vi "SysIdRoutine_Quasistatic.vi"(6 "reset?":bool, 10 "direction":enum16{"kForward", "kReverse"}(ring), 11 "in SysIdRoutine":T3={"m_config"={"m_timeout_Sec"=10.0, "m_stepVoltage_Volt"=7.0, "m_rampRate_V/S"=1.0}, "m_mechanism"={"m_drive_volts"=0.0, "m_log"=[], "m_name"=""}, "m_outputVolts"=0.0, "m_recordState"=enum."kNone", "timer"={"StartTime"=0.0, "Accumulated TIme"=0.0, "Running"=FALSE, "semaphore"=refnum}} {"timer"."Accumulated TIme" format="%13.5p"; "timer"."StartTime" format="%13.5p"}) -> (0 "Expired":bool, 1 "CurrentTimer":dbl, 2 "outputVolts":dbl, 3 "out SysIdRoutine":T3={"m_config"={"m_timeout_Sec"=10.0, "m_stepVoltage_Volt"=7.0, "m_rampRate_V/S"=1.0}, "m_mechanism"={"m_drive_volts"=0.0, "m_log"=[], "m_name"=""}, "m_outputVolts"=0.0, "m_recordState"=enum."kNone", "timer"={"StartTime"=0.0, "Accumulated TIme"=0.0, "Running"=FALSE, "semaphore"=refnum}} {"timer"."Accumulated TIme" format="%13.5p"; "timer"."StartTime" format="%13.5p"})   [LabVIEW 2023]
uses:
  <vilib>/Rock Robotics/WPI/ThirdParty/JAS_Junk/TrajLib/TypeDef/TIMER.ctl
  <vilib>/Utility/semaphor.llb/Obtain Semaphore Reference.vi
  <vilib>/Rock Robotics/WPI/ThirdParty/JAS_Junk/TrajLib/Timer_Reset.vi
  <vilib>/Rock Robotics/WPI/ThirdParty/JAS_Junk/TrajLib/Trajectory_Library.lvlib
panel:
  out "outputSign":dbl
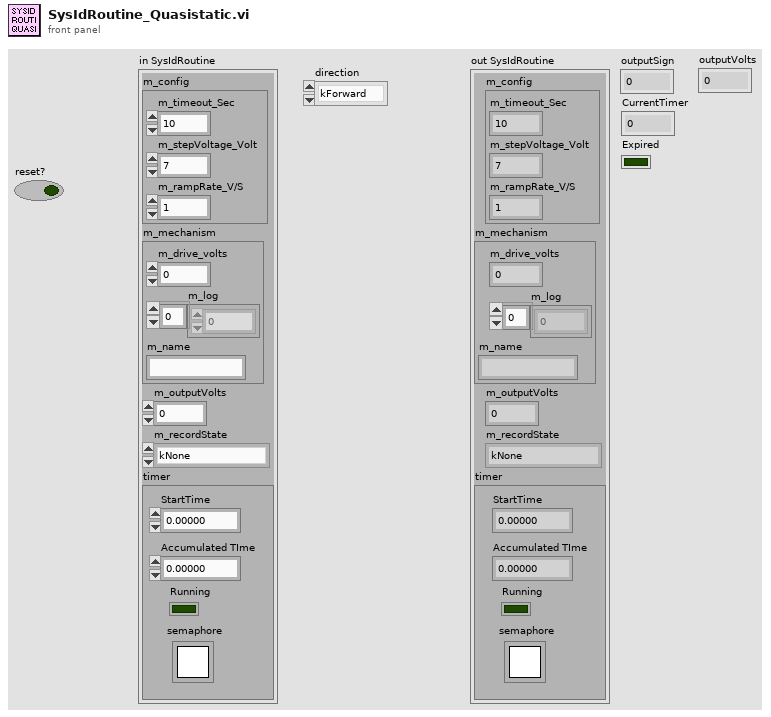
[diagram p1: front panel]
types:
  T1 = typedef "Trajectory_Library.lvlib/TIMER.ctl" = cluster{"StartTime":dbl, "Accumulated TIme":dbl, "Running":bool, "semaphore":T2}
  T2 = typedef "Semaphore RefNum" = refnum<k1>
  T3 = cluster{"m_config":cluster{"m_timeout_Sec":dbl, "m_stepVoltage_Volt":dbl, "m_rampRate_V/S":dbl}, "m_mechanism":cluster{"m_drive_volts":dbl, "m_log":u8[], "m_name":string}, "m_outputVolts":dbl, "m_recordState":enum16{"kQuasistaticForward", "kQuasistaticReverse", "kDynamicForward", "kDynamicReverse", "kNone"}, "timer":T1}
  T4 = enum16{"big-endian, network order", "native, host order", "little-endian"}
  T5 = enum16{"kQuasistaticForward", "kQuasistaticReverse", "kDynamicForward", "kDynamicReverse", "kNone"}
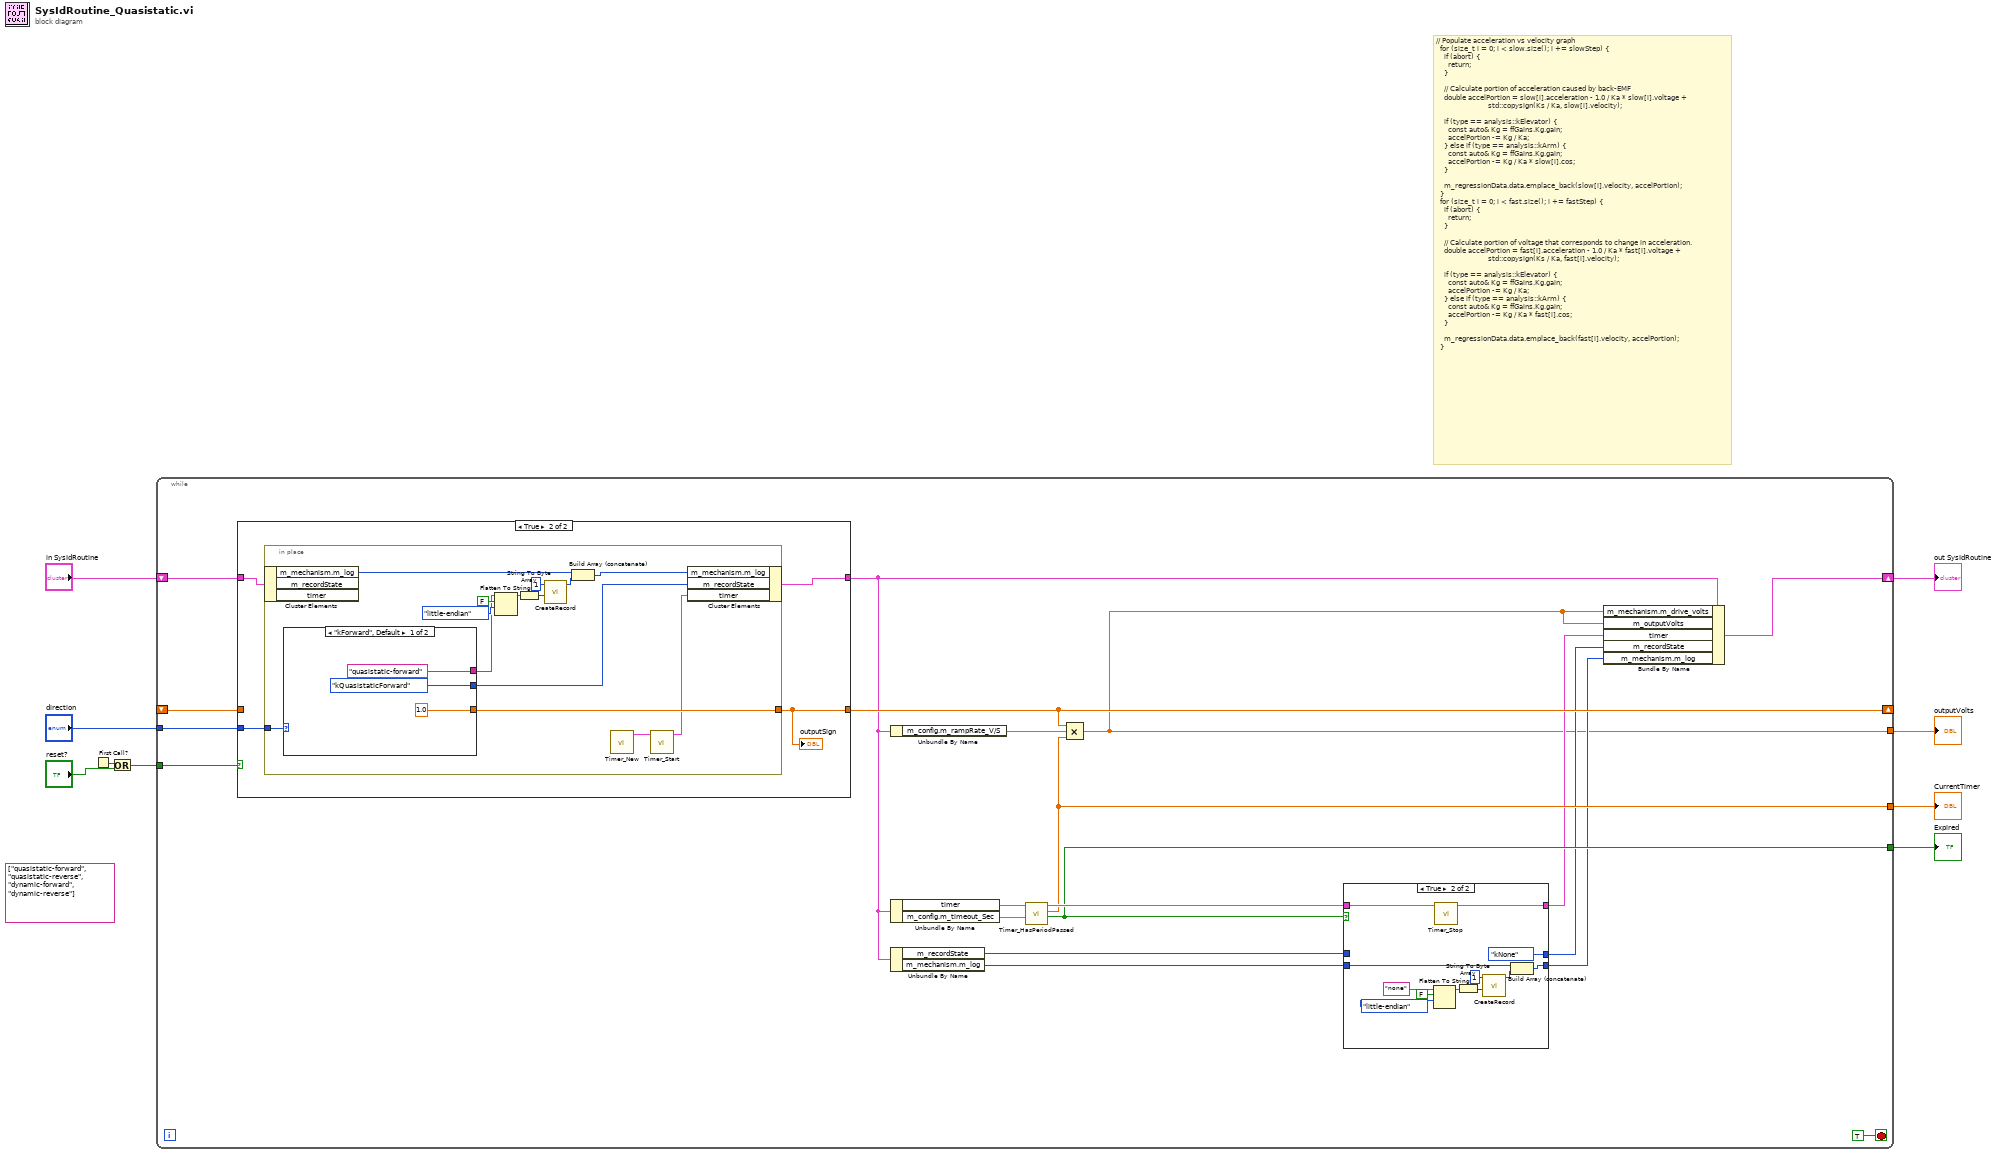
[diagram p0: block diagram]
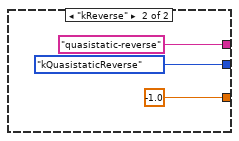
[diagram p3: hidden frame]
diagram:
  (unwired) string[] ["quasistatic-forward", "quasistatic-reverse", "dynamic-forward", "dynamic-reverse"]
  # "// Populate acceleration vs velocity graph\n  for (size_t i = 0; i < slow.size(); i += slowStep) {\n    if (abort) {\n      return;\n    }\n\n    // Calculate portion of acceleration caused by back-EMF\n    double accelPortion = slow[i].acceleration - 1.0 / Ka * slow[i].voltage +\n                          std::copysign(Ks / Ka, slow[i].velocity);\n\n    if (type == analysis::kElevator) {\n      const auto& Kg = ffGains.Kg.gain;\n      accelPortion -= Kg / Ka;\n    } else if (type == analysis::kArm) {\n      const auto& Kg = ffGains.Kg.gain;\n      accelPortion -= Kg / Ka * slow[i].cos;\n    }\n\n    m_regressionData.data.emplace_back(slow[i].velocity, accelPortion);\n  }\n  for (size_t i = 0; i < fast.size(); i += fastStep) {\n    if (abort) {\n      return;\n    }\n\n    // Calculate portion of voltage that corresponds to change in acceleration.\n    double accelPortion = fast[i].acceleration - 1.0 / Ka * fast[i].voltage +\n                          std::copysign(Ks / Ka, fast[i].velocity);\n\n    if (type == analysis::kElevator) {\n      const auto& Kg = ffGains.Kg.gain;\n      accelPortion -= Kg / Ka;\n    } else if (type == analysis::kArm) {\n      const auto& Kg = ffGains.Kg.gain;\n      accelPortion -= Kg / Ka * fast[i].cos;\n    }\n\n    m_regressionData.data.emplace_back(fast[i].velocity, accelPortion);\n  }"
  n1 = First Call?() -> (First Call?: T/F=w4:bool)
  n2 = Or(x=w4, y="reset?") -> (x .or. y?=w2:bool)
  n3 = while {
    tunnel: "direction" -> [w29]
    shift-right: [w23] -> w7
    shift-left: "in SysIdRoutine" -> [w28]
    tunnel: [w21] -> w6
    tunnel: [w20] -> w5
    shift-right: [w19] -> _
    shift-left: _ -> [w18]
    tunnel: w2 -> [w12]
    tunnel: [w11] -> w1
    stop <- TRUE stop-if-true
    n4 = case shown="True" w12 {
      tunnel: w29 -> [_ w35]
      tunnel: w28 -> [w31 w34]
      tunnel: [w30 w33] -> w19
      tunnel: [w31 w32] -> w17
      tunnel: w18 -> [w30 _]
      frame False {
      }
      frame True {
        n5 = in-place {
          in-place-border: w35 -> [w49]
          in-place-border: [w47] -> w33
          n6 = in-place-cluster #1(w34) -> ("m_mechanism.m_log"=w40:u8[])  [unwired: 2 out]
          n7 = case shown="\"kForward\", Default" w49 {
            tunnel: [T5."kQuasistaticForward" ("m_recordState") T5."kQuasistaticReverse" ("m_recordState")] -> w48
            tunnel: [1.0 -1.0] -> w47
            tunnel: ["quasistatic-forward" ("String") "quasistatic-reverse" ("String")] -> w38
            frame "kForward", Default {
            }
            frame "kReverse" {
            }
          }
          n8 = Flatten To String(anything=w38, prepend array or string size? (T)=FALSE, byte order (0:big-endian, network order)=T4."little-endian") -> (data string=w44:string)  [unwired: 1 in, 2 out]
          n9 = String To Byte Array(string=w44) -> (unsigned byte array=w45:u8[])
          n10 = call "CreateRecord.vi"("payload data (little endian)"=w45, "entry ID"=1) -> ("record"=w46:u8[])  [unwired: 9 in]
          n11 = Build Array (concatenate)(w40, w46) -> (w39:u8[])
          n12 = call <vilib>:"Timer_New.vi"() -> ("TIMER"=w37:T1)  [unwired: 11 in]
          n13 = call <vilib>:"Timer_Start.vi"("in Timer"=w37) -> ("out Timer"=w36:T1)  [unwired: 10 in]
          n14 = in-place-cluster #1("m_mechanism.m_log"=w39, "m_recordState"=w48, "timer"=w36) -> (w32:T3)
        }
        "outputSign" <- w33
      }
    }
    n15 = Unbundle By Name(w17) -> ("m_config.m_rampRate_V/S"=w24:dbl)
    n16 = Unbundle By Name(w17) -> ("timer"=w26:T1, "m_config.m_timeout_Sec"=w25:dbl)
    n17 = Unbundle By Name(w17) -> ("m_recordState"=w15:T5, "m_mechanism.m_log"=w10:u8[])
    n18 = call <vilib>:"Timer_HasPeriodPassed.vi"("Period"=w25, "in Timer"=w26) -> ("Expired"=w20:bool, "CurrentTImer"=w21:dbl, "out Timer"=w27:T1)  [unwired: 7 in]
    n19 = Compound Arithmetic op=MULTIPLY(w19, w24, w21) -> (w11:dbl)
    n20 = case shown="True" w20 {
      tunnel: w27 -> [w58 w70]
      tunnel: [w58 w69] -> w16
      tunnel: w10 -> [w57 w61]
      tunnel: [w57 w62] -> w13
      tunnel: [w56 T5."kNone" ("m_recordState")] -> w14
      tunnel: w15 -> [w56 _]
      frame False {
      }
      frame True {
        n21 = Flatten To String(anything="none" ("String"), prepend array or string size? (T)=FALSE, byte order (0:big-endian, network order)=T4."little-endian") -> (data string=w66:string)  [unwired: 1 in, 2 out]
        n22 = call <vilib>:"Timer_Stop.vi"("in Timer"=w70) -> ("out Timer"=w69:T1)  [unwired: 10 in]
        n23 = String To Byte Array(string=w66) -> (unsigned byte array=w67:u8[])
        n24 = call "CreateRecord.vi"("payload data (little endian)"=w67, "entry ID"=1) -> ("record"=w68:u8[])  [unwired: 9 in]
        n25 = Build Array (concatenate)(w61, w68) -> (w62:u8[])
      }
    }
    n26 = Bundle By Name(cluster=w17, "m_mechanism.m_drive_volts"=w11, "m_outputVolts"=w11, "timer"=w16, "m_recordState"=w14, "m_mechanism.m_log"=w13) -> (w23:T3)
  }
  "out SysIdRoutine" <- w7
  "Expired" <- w5
  "CurrentTimer" <- w6
  "outputVolts" <- w1
